vi "Main (control and indicator).vi"() -> ()   [LabVIEW 2009]
doc: "The program uses a Control Reference to give access to a front panel control, to a subVI. The main program calls the subVI. The subVI then writes a random number to the Waveform Chart in the front panel of the main VI. It reads the value from the Boolean control in the main VI front panel to terminate execution of the while loop. The Control References were created by right-clicking on the waveform chart or Boolean terminal and selecting Create > Reference. The Waveform Chart Refnum in the subVI can be created in two ways.\n1. Dragging the Control Reference from the Block Diagram of the Main VI to the Front Panel of the subVI.\n2. Place a Control Refnum of the Front Panel of the subVI by selecting Controls > Refnum > Control Refnum. Then select a Waveform Chart form the Controls palette and drop it inside the Control Refnum Container.\n\nThe Boolean Refnum was created in a similar manner."
panel:
  in  "stop":bool
  out "Waveform Chart":dbl(graph)
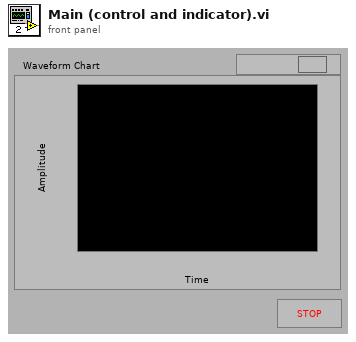
[diagram p1: front panel]
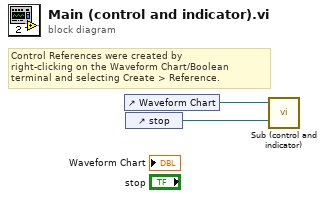
[diagram p0: block diagram]
diagram:
  # "Control References were created by\nright-clicking on the Waveform Chart/Boolean\nterminal and selecting Create > Reference."
  n1 = control-ref of="Waveform Chart"() -> (w2:refnum<vi>)
  n2 = control-ref of="stop"() -> (w1:refnum<vi>)
  n3 = call "Sub (control and indicator).vi"("Bool Refnum"=w1, "WFChart Refnum"=w2) -> ()  [unwired: 1 in]
